vi "fact.vi"(1 "Numeric":dbl=4.0) -> (0 "Fact":dbl=24.0)   [LabVIEW 2013]
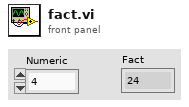
[diagram p1: front panel]
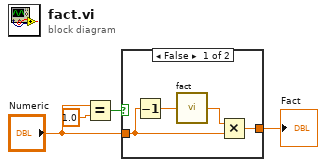
[diagram p0: block diagram]
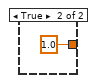
[diagram p2: hidden frame]
diagram:
  n1 = Equal?(x="Numeric", y=1.0) -> (x = y?=w1:bool)
  n2 = case shown="False" w1 {
    tunnel: "Numeric" -> [w6 _]
    tunnel: [w5 1.0] -> w4
    frame False {
      n3 = Decrement(x=w6) -> (x-1=w8:dbl)
      n4 = call "fact.vi"("Numeric"=w8) -> ("Fact"=w7:dbl)
      n5 = Multiply(x=w7, y=w6) -> (x*y=w5:dbl)
    }
    frame True {
    }
  }
  "Fact" <- w4
